vi "TWM Client Recieve Packet.vi"(6 "max message length (1024)":i32=1024, 7 "end of packet key":string="TWM:command:EndOfPacket", 8 "error in":errorcluster, 9 "timeout [ms] (5000 ms)":i32=5000, 10 "message header (empty)":string, 11 "handle in":i32=-1) -> (0 "error out":errorcluster, 2 "message data":string, 3 "handle out":i32)   [LabVIEW 2013, in "TWM Client.lvlib"]
doc: "Receives message from TWM server with timeout. Message is terminated by given key. If header string is passed, the function will check the match with data packet and eventually throw an error."
uses:
  <vilib>/Utility/error.llb/Error Cluster From Error Code.vi
  <vilib>/ErrorRing/Error Ring.xnode
  <vilib>/regexp/Match Regular Expression.xnode
  TWM Client.lvlib
  octave/infolib.lvlibp
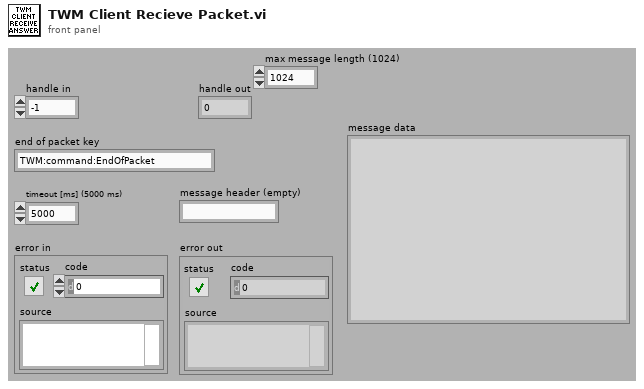
[diagram p1: front panel]
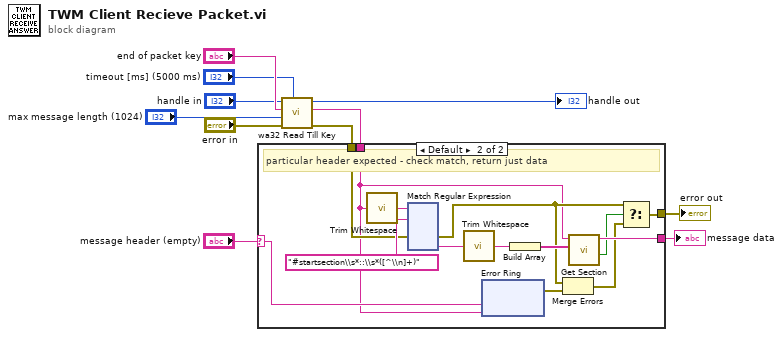
[diagram p0: block diagram]
diagram:
  n1 = call "wa32 Read Till Key.vi"("timeout [ms] (1000)"="timeout [ms] (5000 ms)", "error in"="error in", "max message length (1024)"="max message length (1024)", "key string"="end of packet key", "handle"="handle in") -> ("error out"=w11:errorcluster, "read message"=w5:string, "handle out"=→"handle out":i32)  [unwired: 4 in]
  n2 = case shown="Default" "message header (empty)" {
    selector: "message header (empty)" -> [_ w21]
    tunnel: w11 -> [w12 w25]
    tunnel: w5 -> [w13 w15]
    tunnel: [w13 w22] -> w2
    tunnel: [w12 w16] -> w3
    frame "" {
      # "no header expected - retorn everything"
    }
    frame Default {
      # "particular header expected - check match, return just data"
      n3 = call <vilib>:"Trim Whitespace.vi"("string"=w15) -> ("trimmed string"=w27:string)  [unwired: 1 in]
      n4 = xnode "Match Regular Expression"("input string"=w27, "regular expression"="#startsection\\s*::\\s*([^\\n]+)", "error in"=w25) -> ("error out"=w18:errorcluster, "submatch 1"=w24:string)  [unwired: 3 in, 4 out]
      n5 = call <vilib>:"Trim Whitespace.vi"("string"=w24) -> ("trimmed string"=w14:string)  [unwired: 1 in]
      n6 = xnode "Error Ring"("parameter 0"=w21, "parameter 1"=w15) -> ("error out"=w19:errorcluster)
      n7 = Build Array(w14) -> (w23:string[])
      n8 = Merge Errors(w18, w19) -> (w17:errorcluster)
      n9 = call "Get Section.vi"("sections"=w23, "info data"=w15) -> ("exist"=w20:bool, "section part"=w22:string)  [unwired: 8 in]
      n10 = Select(t=w18, s=w20, f=w17) -> (s? t:f=w16:errorcluster)
    }
  }
  "error out" <- w3
  "message data" <- w2
